vi "B030管理.vi"() -> ()   [LabVIEW 2013]
uses:
  <vilib>/Utility/error.llb/whitespace.ctl
  <vilib>/addons/database/_DB Variant To Data/Database Variant To Data.xnode
panel:
  in  "选项卡控件":enum32{"功能", "输入输出特性"}(tab)
  out "返回":string
  out "表格控件":string[][](table) caption="已注册用户"
  in  "壳体条码":string
  in  "查询":bool
  in  "删除":bool
  in  "合格":bool
  in  "写入":bool
  in  "要写入的条码":string
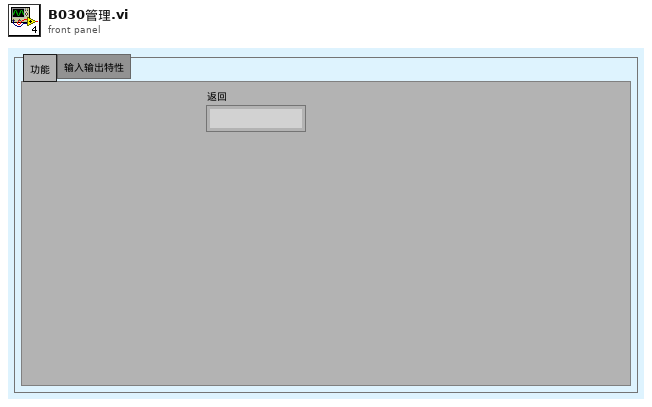
[diagram p1: front panel]
types:
  T1 = enum8{"Enabled", "Disabled", "Disabled and Grayed Out"}
  T2 = cluster{"userCode":string, "userName":string, "userStatus":string, "connectionMode":string, "takesTime":string, "countDone":string, "countOK":string, "countNG":string, "rigStatus":string, "productsName":string, "partCode1":string, "partCode2":string, "partCode3":string}
  T3 = typedef "whitespace.ctl" = u16
  T4 = typedef "LVRowAndColumnTypeDef.ctl" = cluster{"Row":i32, "Column":i32}
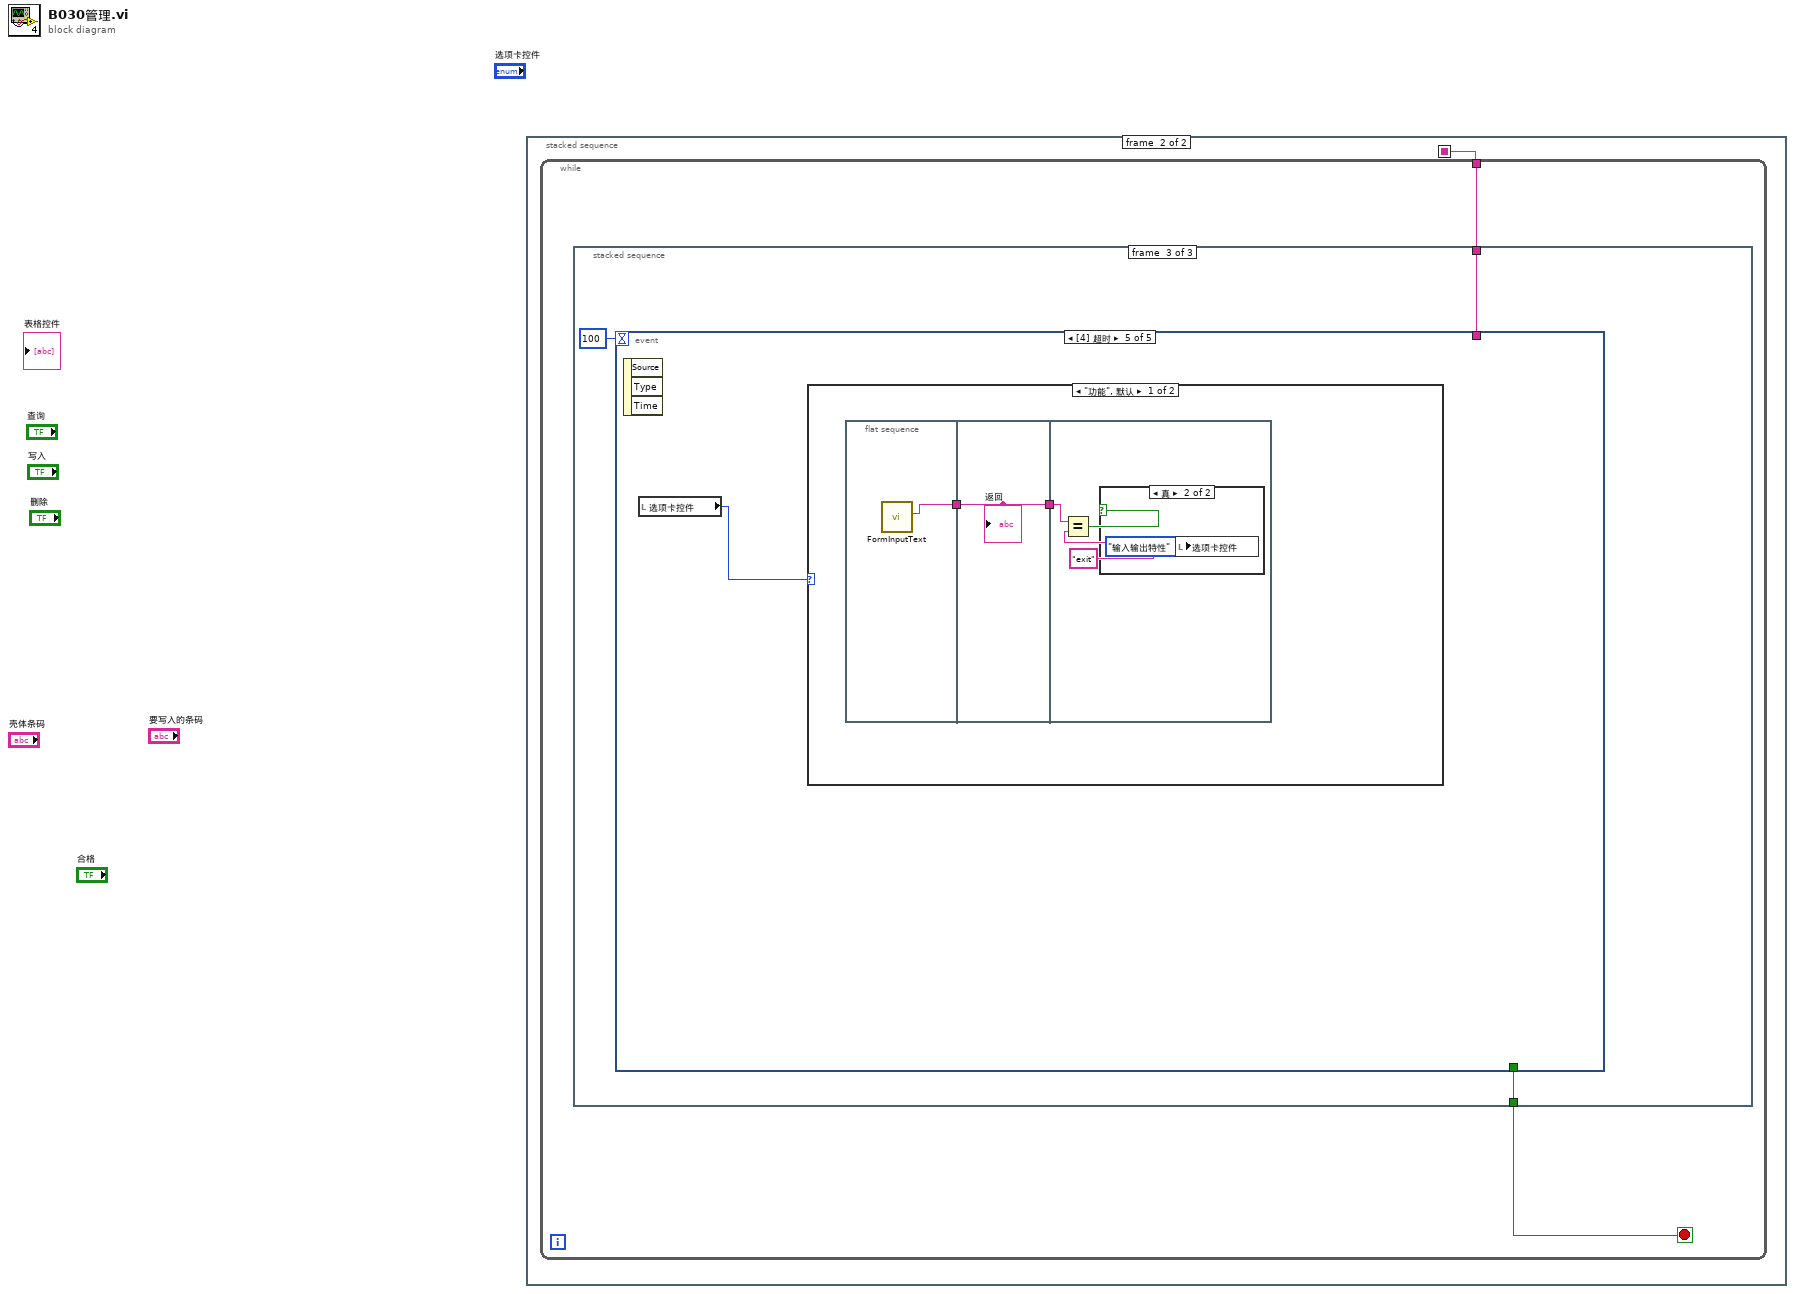
[diagram p0: block diagram]
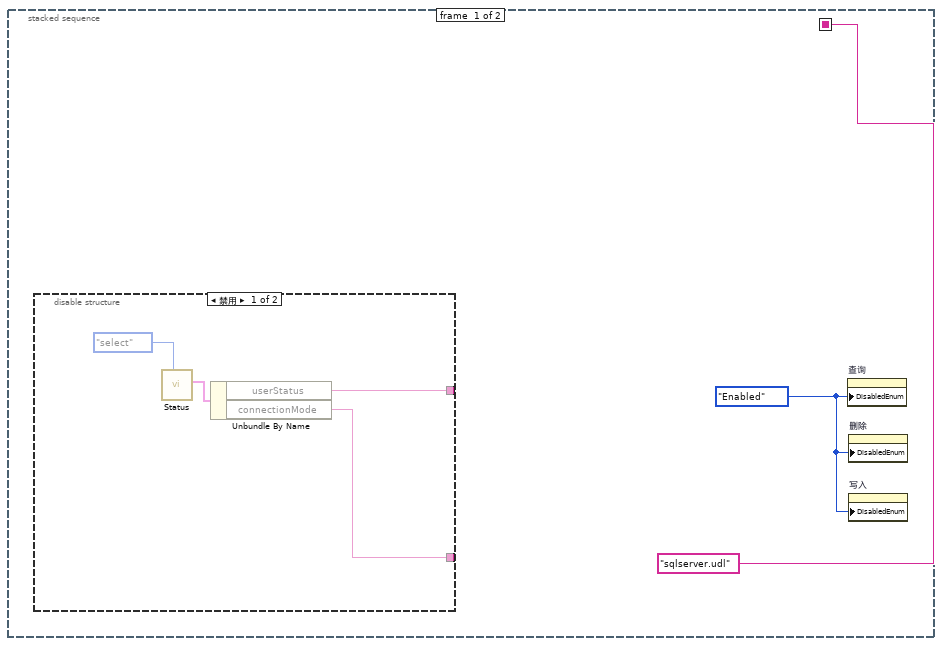
[diagram p2: hidden frame]
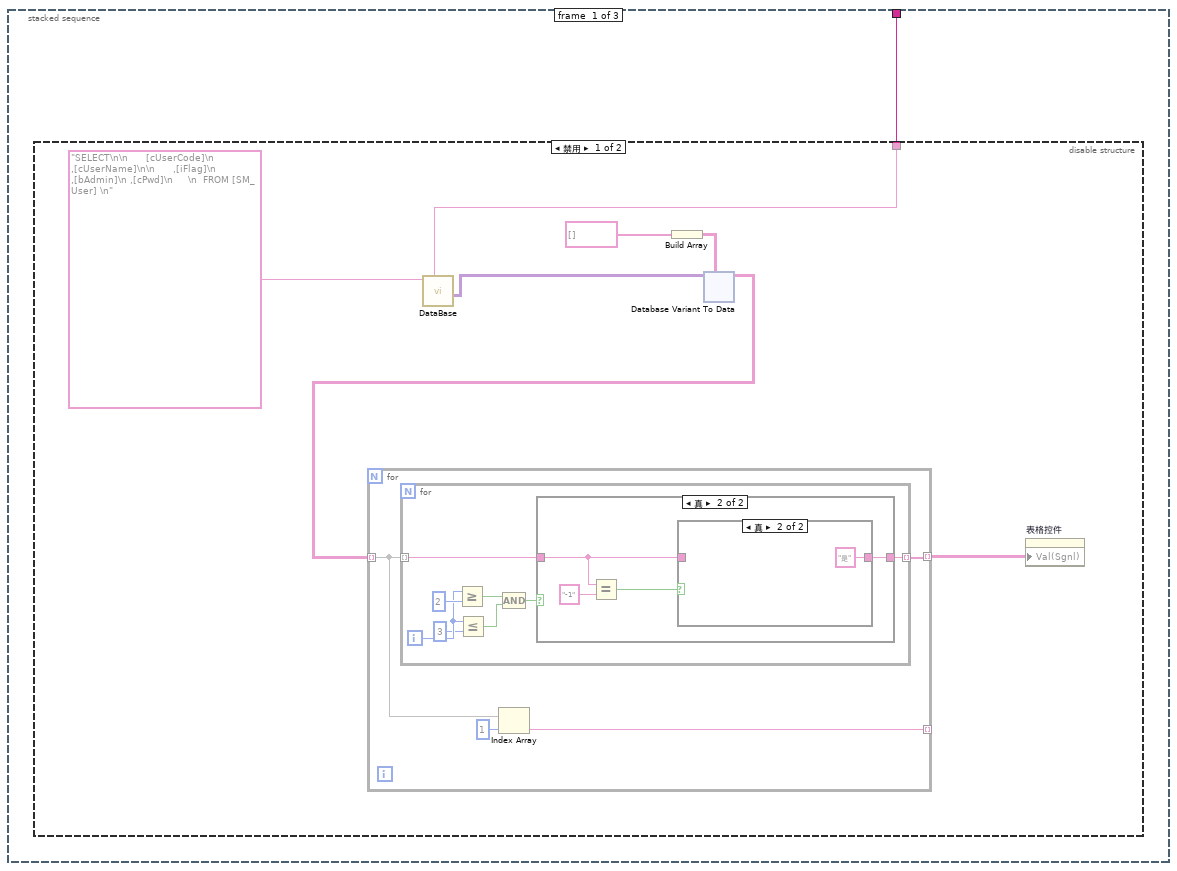
[diagram p4: hidden frame]
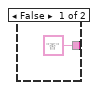
[diagram p6: hidden frame]
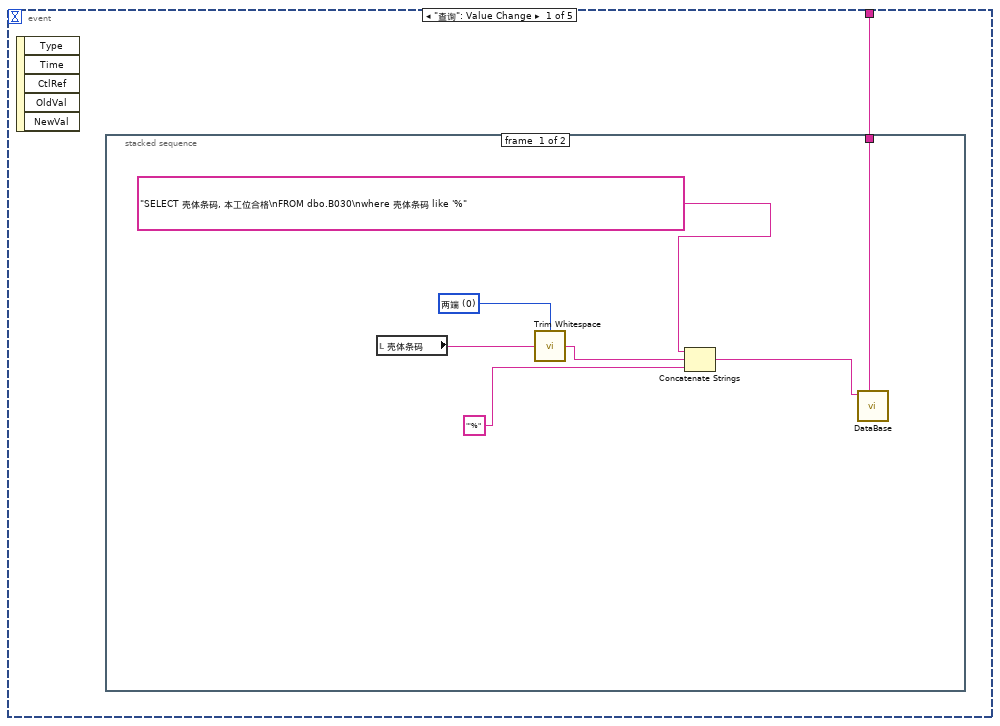
[diagram p9: hidden frame]
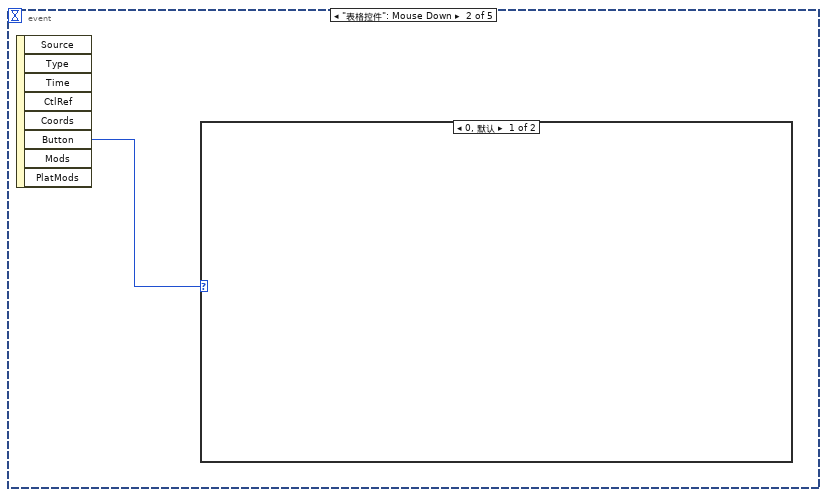
[diagram p11: hidden frame]
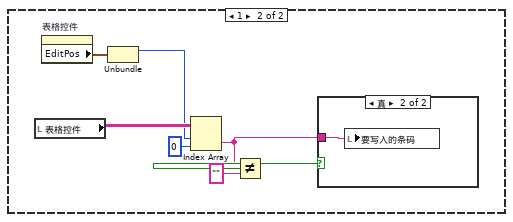
[diagram p12: hidden frame]
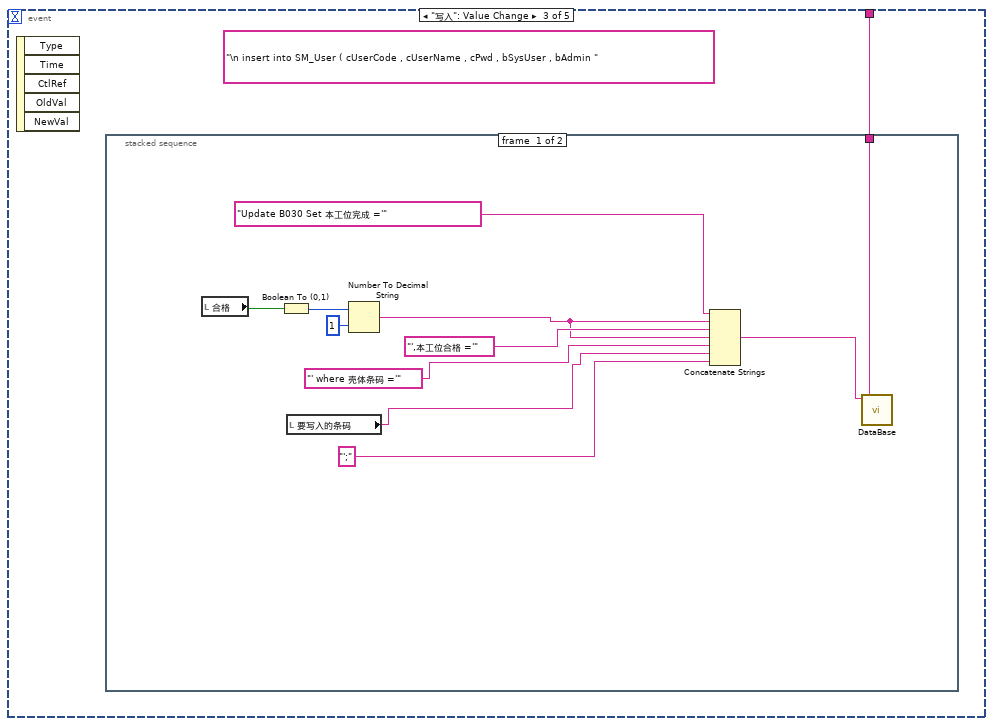
[diagram p14: hidden frame]
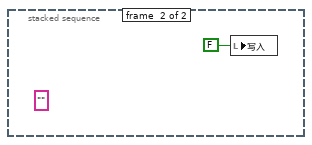
[diagram p15: hidden frame]
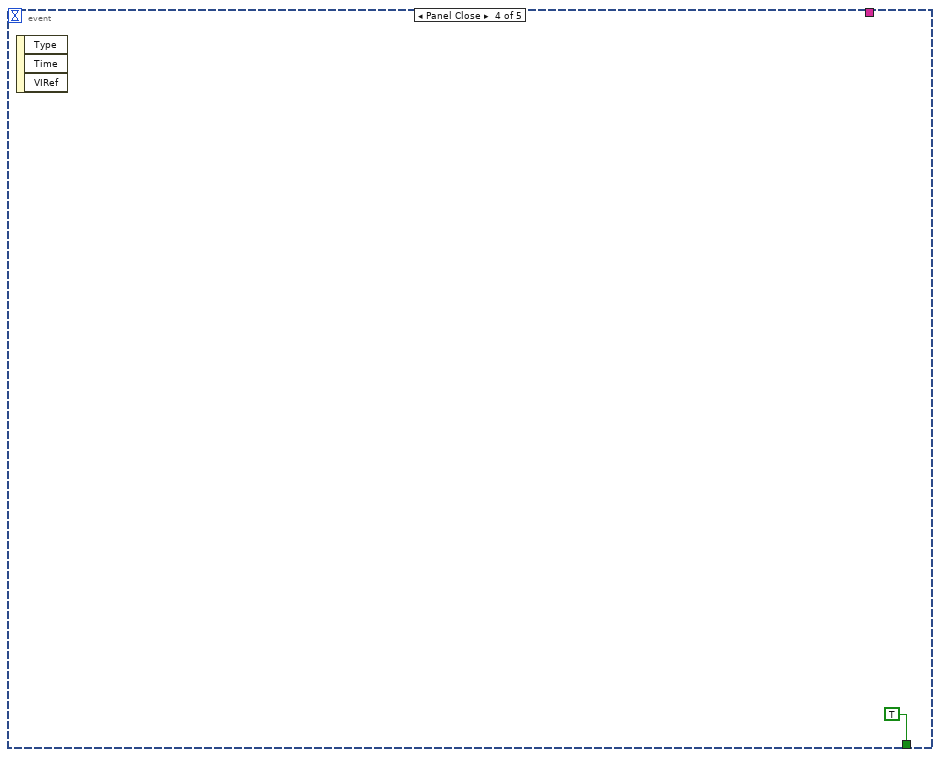
[diagram p16: hidden frame]
diagram:
  n1 = stacked-sequence {
    seq-local: ["sqlserver.udl" ("udl名称") _] -> [_ w7]
    frame #0 {
      w2 = T1."Enabled" ("禁用")
      n2 = disable-structure shown="禁用" {
        disable-tunnel: [w4 _] -> _
        disable-tunnel: [w3 _] -> _
        frame Disabled {
          n3 = call "Status.vi"("模式"=enum16{"select", "insert", "update", "delete"}."select") -> ("元素"=w6:T2)  [unwired: 10 in]
          n4 = Unbundle By Name(w6) -> ("userStatus"=w4:string, "connectionMode"=w3:string)
        }
        frame Enabled {
        }
      }
      n5 = property on="查询" class="Bool (严格)"("DisabledEnum"=w2) -> ()  [unwired: 2 in, 2 out]
      n6 = property on="删除" class="Bool (严格)"("DisabledEnum"=w2) -> ()  [unwired: 2 in, 2 out]
      n7 = property on="写入" class="Bool (严格)"("DisabledEnum"=w2) -> ()  [unwired: 2 in, 2 out]
    }
    frame #1 {
      n8 = while {
        tunnel: w7 -> [w8]
        stop <- w9 stop-if-true
        n9 = stacked-sequence {
          tunnel: [_ _ w83] -> w9
          tunnel: w8 -> [w10 _ w82]
          frame #0 {
            n10 = disable-structure shown="禁用" {
              disable-tunnel: w10 -> [w11 _]
              frame Disabled {
                n11 = call "DataBase.vi"("udl名称"=w11, "SQL query"="SELECT\n\n      [cUserCode]\n      ,[cUserName]\n\n      ,[iFlag]\n      ,[bAdmin]\n ,[cPwd]\n     \n  FROM [SM_User] \n") -> ("recordset data"=w14:variant[][])  [unwired: 9 in]
                n12 = Build Array(string[] [] ("添加的数组")) -> (w15:string[][])
                n13 = xnode ("Database Variant To Data")("database variant"=w14, "type"=w15) -> ("data"=w13:string[][])  [unwired: 1 in, 1 out]
                n14 = for {
                  tunnel: w13 -> [w20] mode=indexing
                  tunnel: [w21] -> w12 mode=indexing
                  tunnel: [w18] -> _ mode=indexing
                  n15 = for {
                    tunnel: w20 -> [w28] mode=indexing
                    tunnel: [w27] -> w21 mode=indexing
                    i -> [w23]
                    n16 = Greater Or Equal?(x=w23, y=2) -> (x >= y?=w25:bool)
                    n17 = Less Or Equal?(x=w23, y=3) -> (x <= y?=w24:bool)
                    n18 = Compound Arithmetic op=AND(w25, w24) -> (w26:bool)
                    n19 = case shown="真" w26 {
                      tunnel: w28 -> [w30 w31]
                      tunnel: [w30 w32] -> w27
                      frame False {
                      }
                      frame True {
                        n20 = Equal?(x=w31, y="-1") -> (x = y?=w33:bool)
                        n21 = case shown="真" w33 {
                          tunnel: ["否" ("字符串") "是" ("字符串")] -> w32
                          tunnel: w31 -> [_ _]
                          frame False {
                          }
                          frame True {
                          }
                        }
                      }
                    }
                  }
                  n22 = Index Array(array=w20, index=1 ("索引")) -> (element=w18:string)
                }
                n23 = property on="表格控件" class="Tbl (严格)"("Val(Sgnl)"=w12) -> ()  [unwired: 2 in, 2 out]
              }
              frame Enabled {
              }
            }
          }
          frame #1 {
          }
          frame #2 {
            n24 = event shown="[4] 超时" {
              selector: _ -> [_ _ _ _ _]
              dyn-events: _ -> [_ _ _ _ _]
              timeout: 100 -> [_ _ _ _ _]
              tunnel: [_ _ _ TRUE _] -> w83
              tunnel: w82 -> [w84 _ w101 _ _]
              event "查询": Value Change {
                n25 = event-data() -> ()  [unwired: 1 in, 5 out]
                n26 = stacked-sequence {
                  tunnel: w84 -> [w91 _]
                  frame #0 {
                    w85 = T3 0 items=["两端", "字符串首端", "字符串末端"] ("location (both)")
                    n27 = local read "壳体条码"() -> (w87:string)
                    n28 = call <vilib>:"Trim Whitespace.vi"("string"=w87, "location (both)"=w85) -> ("trimmed string"=w86:string)
                    n29 = Concatenate Strings("SELECT 壳体条码, 本工位合格\nFROM dbo.B030\nwhere 壳体条码 like '%" ("SQL query"), w86, "'%") -> (w88:string)
                    n30 = call "DataBase.vi"("udl名称"=w91, "SQL query"=w88) -> ()  [unwired: 9 in, 1 out]
                  }
                  frame #1 {
                  }
                }
              }
              event "表格控件": Mouse Down {
                n31 = event-data() -> ("Button"=w92:u16)  [unwired: 1 in, 7 out]
                n32 = case shown="0, 默认" w92 {
                  frame 0, Default {
                  }
                  frame 1 {
                    n33 = local read "表格控件"() -> (w98:string[][])
                    n34 = property on="表格控件" class="Tbl (严格)"() -> ("EditPos"=w99:T4)  [unwired: 2 in, 2 out]
                    n35 = Unbundle(w99) -> ("Row"=w97:i32)  [unwired: 1 out]
                    n36 = Index Array(array=w98, index (row)=w97, index (col)=0 ("禁用的索引 (列)")) -> (element=w93:string)
                    n37 = Not Equal?(x=w93, y="") -> (x != y?=w94:bool)
                    n38 = case shown="真" w94 {
                      tunnel: w93 -> [_ w100]
                      frame False {
                      }
                      frame True {
                        n39 = local write "要写入的条码"(w100) -> ()
                      }
                    }
                  }
                }
              }
              event "写入": Value Change {
                (unwired) "\n insert into SM_User ( cUserCode , cUserName , cPwd , bSysUser , bAdmin " ("SQL query")
                n40 = event-data() -> ()  [unwired: 1 in, 5 out]
                n41 = stacked-sequence {
                  tunnel: w101 -> [w112 _]
                  frame #0 {
                    n42 = local read "合格"() -> (w111:bool)
                    n43 = Boolean To (0,1)(Boolean=w111) -> (0, 1=w110:i16)
                    n44 = local read "要写入的条码"() -> (w104:string)
                    n45 = Number To Decimal String(number=w110, width (-)=i16 1 ("宽度(-)")) -> (decimal integer string=w106:string)
                    n46 = Concatenate Strings("Update B030 Set 本工位完成 ='" ("SQL query"), w106, "',本工位合格 ='", w106, "' where 壳体条码 ='", w104, "';") -> (w102:string)
                    n47 = call "DataBase.vi"("udl名称"=w112, "SQL query"=w102) -> ()  [unwired: 9 in, 1 out]
                  }
                  frame #1 {
                    (unwired) ""
                    n48 = local write "写入"(FALSE ("注册")) -> ()
                  }
                }
              }
              event Panel Close {
                n49 = event-data() -> ()  [unwired: 1 in, 3 out]
              }
              event Timeout {
                n50 = event-data() -> ()  [unwired: 1 in, 3 out]
                n51 = local read "选项卡控件"() -> (w115:enum32{"功能", "输入输出特性"})
                n52 = case shown="\"功能\", 默认" w115 {
                  frame "功能", Default {
                    n53 = flat-sequence {
                      tunnel: [w118] -> w116
                      tunnel: [w119] -> w117
                      tunnel: w116 -> [w119]
                      tunnel: w117 -> [w122]
                      frame #0 {
                        n54 = call "FormInputText.vi"() -> ("返回"=w118:string)  [unwired: 11 in]
                      }
                      frame #1 {
                        "返回" <- w119
                      }
                      frame #2 {
                        n55 = Equal?(x=w122, y="exit") -> (x = y?=w120:bool)
                        n56 = case shown="真" w120 {
                          frame False {
                          }
                          frame True {
                            n57 = local write "选项卡控件"(enum32{"功能", "输入输出特性", "电流特性"}."输入输出特性" ("选项卡控件")) -> ()
                          }
                        }
                      }
                    }
                  }
                  frame "输入输出特性" {
                  }
                }
              }
            }
          }
        }
      }
    }
  }
